vi "coag pump.vi"(6 "Coagulant control":T1, 10 "coagulant dose [mg/L]":dbl, 11 "plant flow [L/s]":dbl) -> (1 "coag dose [mg/L]":dbl, 2 "pump [V]":dbl, 3 "coagulant flow [mL/s]":dbl)   [LabVIEW 2014]
uses:
  ProCoDA/DAQ configuration/Sensor buffer command.ctl
  Manual or Auto.ctl
panel:
  in  "coagulant stock [g/L]":dbl=72.0
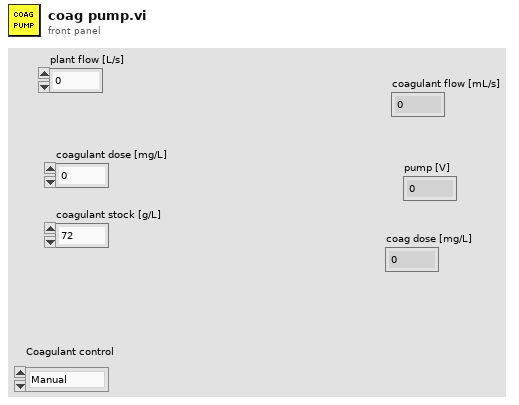
[diagram p1: front panel]
types:
  T1 = typedef "Manual or Auto.ctl" = enum16{"Manual", "Automatic"}
  T2 = typedef "Sensor buffer command.ctl" = enum16{"set buffer size", "write", "refill buffer", "read recent", "read all", "clear"}
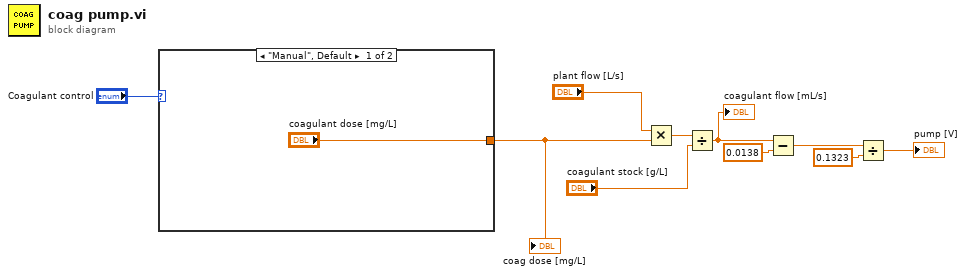
[diagram p0: block diagram]
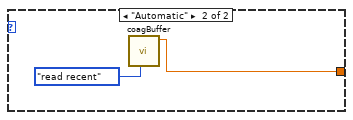
[diagram p2: hidden frame]
diagram:
  n1 = case shown="\"Manual\", Default" "Coagulant control" {
    tunnel: ["coagulant dose [mg/L]" w12] -> w1
    frame "Manual", Default {
    }
    frame "Automatic" {
      n2 = call "coagBuffer.vi"("command"=Sensor_buffer_command."read recent") -> ("recent coag"=w12:dbl)  [unwired: 8 in, 2 out]
    }
  }
  "coag dose [mg/L]" <- w1
  n3 = Multiply(x="plant flow [L/s]", y=w1) -> (x*y=w9:dbl)
  n4 = Divide(x=w9, y="coagulant stock [g/L]") -> (x/y=w6:dbl)
  "coagulant flow [mL/s]" <- w6
  n5 = Subtract(x=w6, y=0.0138) -> (x-y=w5:dbl)
  n6 = Divide(x=w5, y=0.1323) -> (x/y=→"pump [V]":dbl)
